vi "Get Components Directory.vi"(8 "error in (no error)":errorcluster, 11 "Framework in":refnum<class "Framework.lvclass">) -> (0 "error out":errorcluster, 2 "components directory":path, 3 "Framework out":refnum<class "Framework.lvclass">)   [LabVIEW 2017, in "DSF Core.lvlib" / "Framework.lvclass"]
uses:
  Framework.lvclass
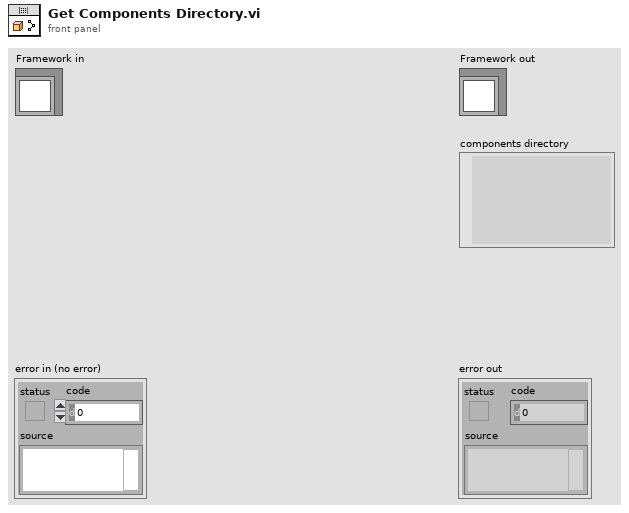
[diagram p1: front panel]
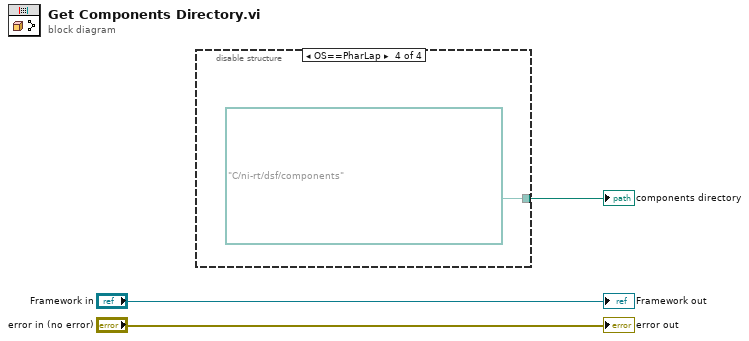
[diagram p0: block diagram]
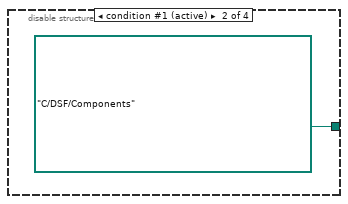
[diagram p3: hidden frame]
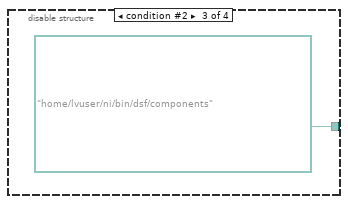
[diagram p4: hidden frame]
diagram:
  n1 = disable-structure shown="OS==PharLap" {
    disable-tunnel: [_ path "C:/DSF/Components" ("transceivers directory") path "/home/lvuser/ni/bin/dsf/components" ("transceivers directory") path "C:/ni-rt/dsf/components" ("transceivers directory")] -> w1
    frame condition #0 {
    }
    frame condition #1 (active) {
    }
    frame condition #2 {
    }
    frame condition #3 {
    }
  }
  "components directory" <- w1
  "error out" <- "error in (no error)"
  "Framework out" <- "Framework in"
